vi "DetectBalls.vi"() -> ()   [LabVIEW 2015]
uses:
  <vilib>/Platform/TimedLoop/XDataNode/timing_clust.ctl
  <vilib>/Platform/TimedLoop/XDataNode/nitl_modes.ctl
  <vilib>/Platform/TimedLoop/XDataNode/wakeup.ctl
  <vilib>/vision/Image Controls.llb/IMAQ Image.ctl
  <vilib>/Platform/TimedLoop/XDataNode/XDataNode.xnode
  <vilib>/Platform/TimedLoop/XDataNode/XDNodeRunTimeDep.lvlib
  <resource>/objmgr/IMAQImage.rc
panel:
  in  "Tracking treshold":i32=40
  out "Speed (px/frame)":i32
  out "Out of Border":bool
  out "Circles Data (Circle Detection 1)":T1(array[cluster])
  in  "Min Radius (Circle Detection 1)":sgl=15.0
  in  "Reset":bool
  in  "Snap":bool
  out "Camera Image":T2(plugin-control)
  out "Snap":T2(plugin-control)
  out "Detection":T2(plugin-control)
  in  "Stop (F)":bool
  # "TEACHING"
  # "Settings"
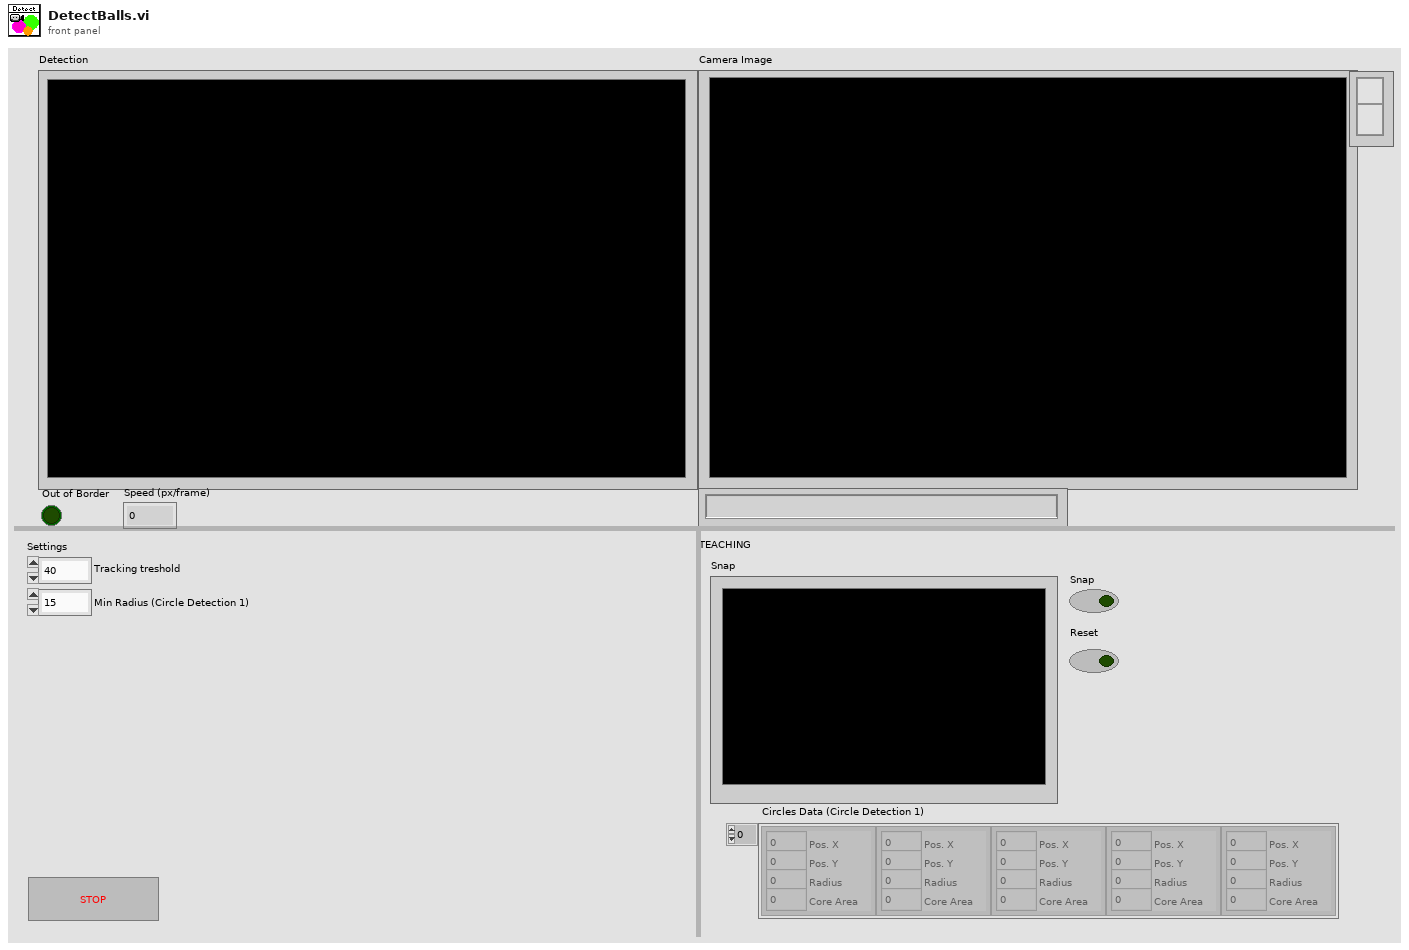
[diagram p1: front panel]
types:
  T1 = cluster{"Pos. X":i32, "Pos. Y":i32, "Radius":i32, "Core Area":i32}[]
  T2 = typedef "IMAQ Image.ctl" = refnum<image>
  T3 = typedef "XDNodeRunTimeDep.lvlib/timing_clust.ctl" = cluster{"Expected End [f-1]":u64, "Actual End [f-1]":u64, "Finished Late? [f-1]":bool, "Expected End [i-1]":u64, "Actual End [i-1]":u64, "Finished Late? [i-1]":bool, "Expected Start [i]":u64, "Actual Start [i]":u64, "Expected Start [f]":u64, "Actual Start [f]":u64, "Source Name":string, "Structure Name":string, "Period":i64, "Deadline":i64, "Offset":i64, "Start":i64, "Priority":i32, "Timeout":i32, "Mode":T4, "Wakeup Reason":T5, "Error":errorcluster, "Source Type":string, "Secondary Source Type":string, "Global End Time":u64, "Global Start Time":u64, "Frame Duration":u64, "Iteration Duration":u64, "Assigned CPU":i32, "I/O Scan Engine Mode":u32}
  T4 = typedef "XDNodeRunTimeDep.lvlib/nitl_modes.ctl" = enum32{"No Change", "Process missed periods, maintain original phase", "Discard missed periods, maintain original phase", "Process missed periods, ignore original phase", "Discard missed periods, ignore original phase"}
  T5 = typedef "XDNodeRunTimeDep.lvlib/wakeup.ctl" = enum32{"Normal", "Aborted", "Asynchronous wakeup", "Timing source error", "Timed loop error", "Timeout"}
  T6 = cluster{"Global Rectangle":i32[], "Contours":cluster{"Contour Type":u32, "ROI Type":u32, "Points":i32[]}[]}
  T7 = cluster{"dXY":i32, "Pos. X":i32, "Pos. Y":i32, "Radius":i32, "Core Area":i32}
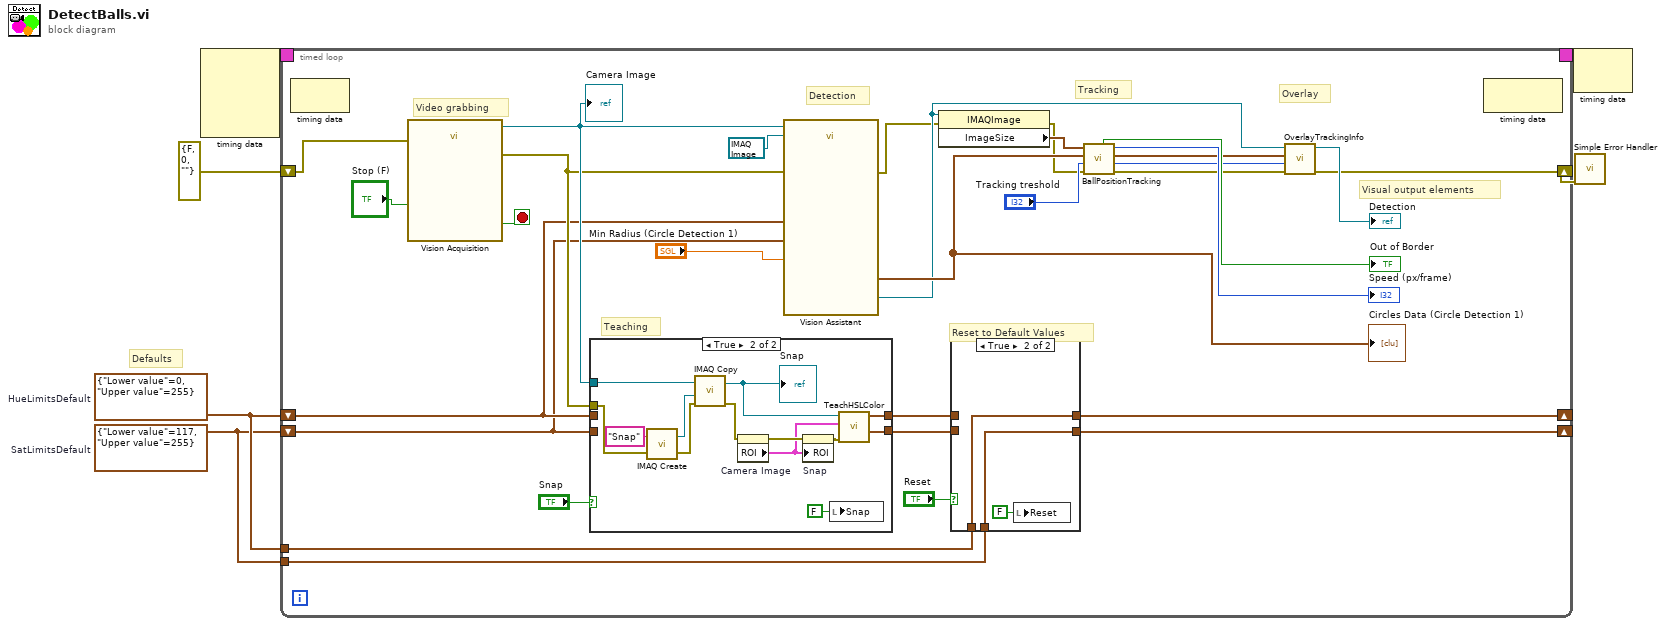
[diagram p0: block diagram]
diagram:
  w5 = cluster{"Lower value":u8, "Upper value":u8} {"Lower value"=117, "Upper value"=255}  # SatLimitsDefault
  w6 = cluster{"Lower value":u8, "Upper value":u8} {"Lower value"=0, "Upper value"=255}  # HueLimitsDefault
  # "Defaults"
  n1 = node-c288() -> (w4:T3)  [unwired: 4 in]
  n2 = timed-loop {
    shift-right: [w30] -> _
    shift-left: w6 -> [w28]
    tunnel: w6 -> [w27]
    shift-right: [w25] -> _
    shift-left: w5 -> [w23]
    tunnel: w5 -> [w24]
    timing: w4 -> [_]
    timing-out: [_] -> w3
    shift-right: [w8] -> w1
    shift-left: errorcluster {"status"=FALSE, "code"=0, "source"=""} ("error out") -> [w7]
    stop <- w35 stop-if-true
    # "Visual output elements"
    # "Overlay"
    # "Tracking"
    # "Reset to Default Values"
    # "Video grabbing"
    # "Teaching"
    # "Detection"
    n3 = node-c288() -> ()  [unwired: 1 in, 1 out]
    n4 = call "Vision Acquisition"("Stop (F)"="Stop (F)", "error in"=w7) -> ("Image Out"=w34:T2, "Stopped"=w35:bool, "error out"=w33:errorcluster)  [unwired: 22 in, 1 out]
    "Camera Image" <- w34
    n5 = case shown="True" "Snap" {
      tunnel: w34 -> [_ w58]
      tunnel: w33 -> [_ w52]
      tunnel: [w45 w50] -> w29
      tunnel: w28 -> [w45 _]
      tunnel: [w44 w49] -> w26
      tunnel: w23 -> [w44 _]
      frame False {
      }
      frame True {
        n6 = call "IMAQ Create"("Image Name"="Snap", "error in (no error)"=w52) -> ("New Image"=w53:T2, "error out"=w51:errorcluster)  [unwired: 3 in]
        n7 = call "IMAQ Copy"("error in (no error)"=w51, "Image Dst"=w53, "Image Src"=w58) -> ("error out"=w47:errorcluster, "Image Dst Out"=w55:T2)  [unwired: 3 in]
        "Snap" <- w55
        n8 = property on="Camera Image" class="ImageControl"(error in=w47) -> (error out=w48:errorcluster, "ROI"=w46:T6)  [unwired: 1 in, 1 out]
        n9 = property on="Snap" class="ImageControl"(error in=w48, "ROI"=w46) -> (error out=w56:errorcluster)  [unwired: 1 in, 1 out]
        n10 = local write "Snap"(FALSE ("Snap")) -> ()
        n11 = call "TeachHSLColor.vi"("error in (no error)"=w56, "ROI Descriptor"=w46, "Image in"=w55) -> ("SatLimits"=w49:cluster{"Lower value":u8, "Upper value":u8}, "HueLimits"=w50:cluster{"Lower value":u8, "Upper value":u8})  [unwired: 5 in, 1 out]
      }
    }
    n12 = call "Vision Assistant"("Image In"=w34, "Image Dst"=T2 refnum, "Red or Hue Range (Color Threshold 1)"=w28, "Green or Sat Range (Color Threshold 1)"=w23, "Min Radius (Circle Detection 1)"="Min Radius (Circle Detection 1)", "error in"=w33) -> ("Image Out"=w12:T2, "Circles Data (Circle Detection 1)"=w22:T1, "error out"=w10:errorcluster)  [unwired: 19 in]
    "Circles Data (Circle Detection 1)" <- w22
    n13 = property class="IMAQImage"(reference=w12, error in=w10) -> (error out=w9:errorcluster, "ImageSize"=w13:cluster{"x":i32, "y":i32})  [unwired: 1 out]
    n14 = case shown="True" "Reset" {
      tunnel: [w40 w43] -> w30
      tunnel: w29 -> [w40 _]
      tunnel: w27 -> [_ w43]
      tunnel: w26 -> [w39 _]
      tunnel: [w39 w42] -> w25
      tunnel: w24 -> [_ w42]
      frame False {
      }
      frame True {
        n15 = local write "Reset"(FALSE ("Reset")) -> ()
      }
    }
    n16 = call "BallPositionTracking.vi"("error in (no error)"=w9, "Tracking treshold"="Tracking treshold", "Circles Data"=w22, "Screen Dimensions"=w13) -> ("error out"=w14:errorcluster, "maxDistance"=w15:i32, "Ball Tracking Position Data"=w16:T7, "Speed"=→"Speed (px/frame)":i32, "OOB"=→"Out of Border":bool)  [unwired: 3 in]
    n17 = call "OverlayTrackingInfo.vi"("error in (no error)"=w14, "maxDistance"=w15, "Ball Tracking Position Data"=w16, "Image in"=w12) -> ("error out"=w8:errorcluster, "Processed Image Out"=→"Detection":T2)  [unwired: 6 in]
    n18 = node-c288() -> ()  [unwired: 1 in, 1 out]
  }
  n19 = node-c288(w3) -> ()  [unwired: 1 out]
  n20 = call <vilib>:"Simple Error Handler.vi"("error in (no error)"=w1) -> ()  [unwired: 4 in, 5 out]
